vi "SDG60OutputOnOff.vi"(2 "error in (no error)":errorcluster, 3 "Enable Output (T: Enable)":bool=TRUE, 4 "Channel (1: Channel1)":u16(ring)=1 items=["Channel1"=1, "Channel2"=2], 5 "VISA resource name":refnum<visa-resource-name>="USB0::0xF4EC::0x1101::SDG6XEBC5R0119::INSTR") -> (0 "error out":errorcluster, 1 "VISA resource name out":refnum<visa-resource-name>)   [LabVIEW 2018]
doc: "Configures the output impedance and source impedance for the channel you specify."
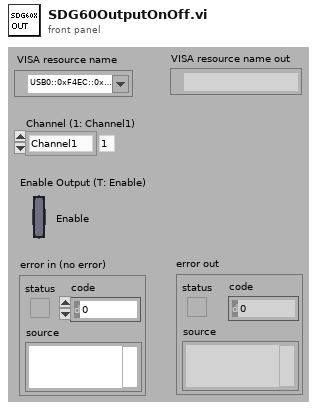
[diagram p1: front panel]
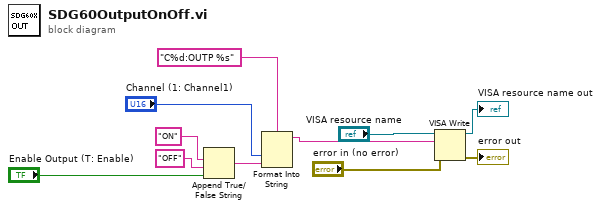
[diagram p0: block diagram]
diagram:
  n1 = Append True/False String(1:"Enable Output (T: Enable)", 2:"OFF" ("true string"), 3:"ON" ("true string")) -> (0:w2:string)  [unwired: 1 in]
  n2 = Format Into String(format string="C%d:OUTP %s", "Channel (1: Channel1)", w2) -> (resulting string=w1:string)  [unwired: 2 in, 1 out]
  n3 = VISA Write(VISA resource name="VISA resource name", write buffer=w1, error in (no error)="error in (no error)") -> (VISA resource name out=→"VISA resource name out":refnum<visa-resource-name>, error out=→"error out":errorcluster)  [unwired: 1 out]
